vi "WriteFGVError.vi"(8 "error in (no error)":errorcluster, 10 "0Cv/1St":i32, 11 "LineScan in":refnum<class "LineScan.lvclass">) -> (0 "error out":errorcluster, 3 "LineScan out":refnum<class "LineScan.lvclass">)   [LabVIEW 2019, in "LineScan.lvclass"]
uses:
  LineScan.lvclass
  Ctrl/Auto Inspection Data Name.ctl
  Ctrl/Auto Inspection Station Name2.ctl
  98c3ab18-6b48-4e70-9579-4f92e907e1f5.vi
  <vilib>/JDP Science/JSONtext/Variant to JSON Text.vi
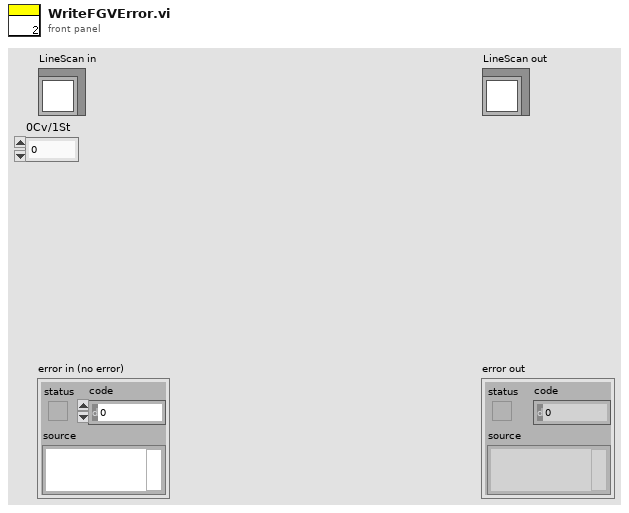
[diagram p1: front panel]
types:
  T1 = typedef "Auto Inspection Data Name.ctl" = enum16{"LocalRun", "ItemSN(TimeCode)", "CurrentAction", "Error", "Data", "OKNG", "電壓值", "電壓值判斷", "電流值", "電流值判斷", "Laser1 Data", "Laser2 Data", "Laser OKNG", "StationNO"}
  T2 = typedef "Auto Inspection Station Name2.ctl" = enum16{"S1Barcode", "S2Measure", "S3Measure", "S4Measure", "S5Measure", "S11_LaserCheck", "S8_Vision AI"}
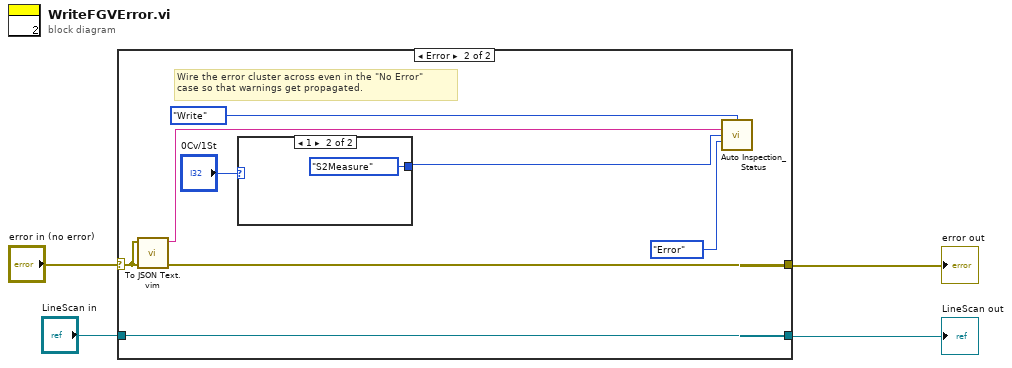
[diagram p0: block diagram]
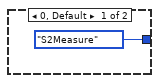
[diagram p3: hidden frame]
diagram:
  n1 = case shown="Error" "error in (no error)" {
    selector: "error in (no error)" -> [w6 w9]
    tunnel: [w6 w9] -> w1
    tunnel: [w5 w13] -> w3
    tunnel: "LineScan in" -> [w5 w13]
    frame No Error {
    }
    frame Error {
      # "Wire the error cluster across even in the \"No Error\"\ncase so that warnings get propagated."
      n2 = call "To JSON Text.vim"("Anything"=w9) -> ("<JSON>"=w10:string)  [unwired: 9 in, 1 out]
      n3 = case shown="1" "0Cv/1St" {
        tunnel: [Auto_Inspection_Station_Name2."S2Measure" ("Station") Auto_Inspection_Station_Name2."S2Measure" ("Station")] -> w7
        frame 0, Default {
        }
        frame 1 {
        }
      }
      n4 = call "Auto Inspection_Status.vi"("Action"=enum16{"Initial", "Write", "Read"}."Write", "DataIn"=w10, "Station"=w7, "Data"=Auto_Inspection_Data_Name."Error") -> ()  [unwired: 9 in, 3 out]
    }
  }
  "error out" <- w1
  "LineScan out" <- w3
